vi "DAC.vi"() -> ()   [LabVIEW 2017]
panel:
  out "Array 4":u32[](array[numeric]) format="%x"
  out "Array 3":u32[](array[numeric]) format="%x"
  out "Array 2":u32[](array[numeric]) format="%x"
  out "Array":u32[](array[numeric]) format="%x"
  in  "SMA mode":bool
  in  "Thresholds (mV)":u16[](array[numeric])=[580, 580, 600, 600, 600, 600, 600, 600]
  in  "Thresholds":u16=600
  in  "one key for threshold":bool
  in  "address":string="192.168.10.10"
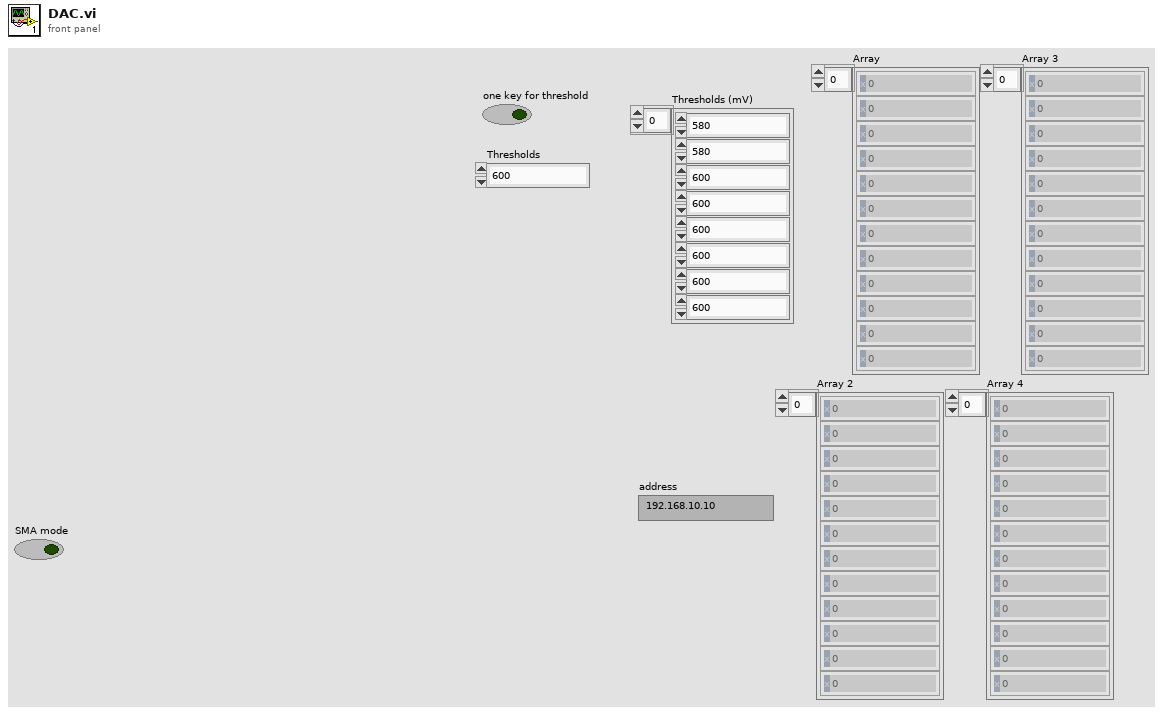
[diagram p1: front panel]
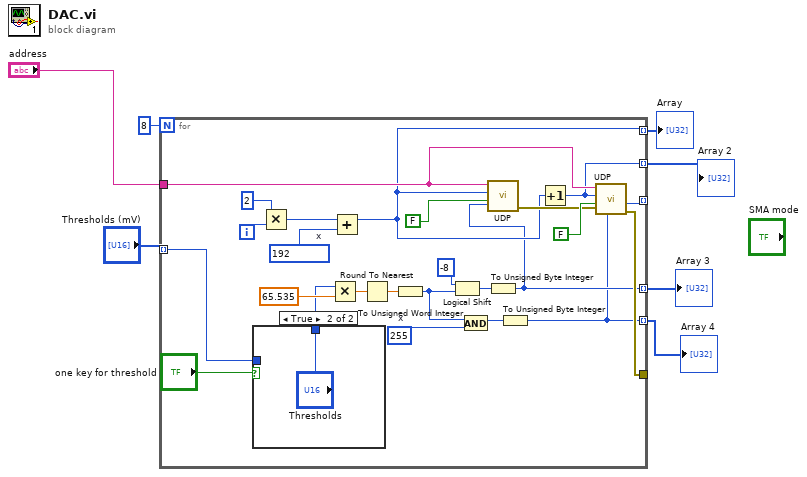
[diagram p0: block diagram]
diagram:
  n1 = for {
    N: 8 -> [_]
    tunnel: "address" -> [w26]
    tunnel: "Thresholds (mV)" -> [w13] mode=indexing
    tunnel: [w21] -> _ mode=indexing
    tunnel: [w16] -> _
    tunnel: [w11] -> w4 mode=indexing
    tunnel: [w10] -> w3 mode=indexing
    tunnel: [w9] -> w2 mode=indexing
    tunnel: [w8] -> w1 mode=indexing
    i -> [w32]
    w12 = u16 192  # x
    w23 = u16 255  # x
    n2 = case shown="True" "one key for threshold" {
      tunnel: [w33 "Thresholds"] -> w14
      tunnel: w13 -> [w33 _]
      frame False {
      }
      frame True {
      }
    }
    n3 = Multiply(x=2, y=w32) -> (x*y=w17:i32)
    n4 = Multiply(x=w14, y=65.535) -> (x*y=w29:dbl)
    n5 = Add(x=w17, y=w12) -> (x+y=w11:i32)
    n6 = Round To Nearest(number=w29) -> (nearest integer value=w27:dbl)
    n7 = To Unsigned Word Integer(number=w27) -> (unsigned 16bit integer=w19:u16)
    n8 = Logical Shift(y=i16 -8, x=w19) -> (x << y=w24:u16)
    n9 = And(x=w19, y=w23) -> (x .and. y?=w22:u16)
    n10 = To Unsigned Byte Integer(number=w24) -> (unsigned 8bit integer=w9:u8)
    n11 = call "UDP.vi"("In"=w9, "Read (TRUE)"=FALSE, "Address"=w11, "IP address"=w26) -> ("error out"=w18:errorcluster)  [unwired: 5 in, 1 out]
    n12 = To Unsigned Byte Integer(number=w22) -> (unsigned 8bit integer=w8:u8)
    n13 = Increment(x=w11) -> (x+1=w10:i32)
    n14 = call "UDP.vi"("In"=w8, "error in (no error)"=w18, "Read (TRUE)"=FALSE, "Address"=w10, "IP address"=w26) -> ("error out"=w16:errorcluster, "Out"=w21:u8)  [unwired: 4 in]
  }
  "Array" <- w4
  "Array 2" <- w3
  "Array 3" <- w2
  "Array 4" <- w1
